vi "2nd head(json).vi"(11 "value":string[](array[string])=["@secondNumber@", "@itemName@", "@startTime@", "@stopTime@", "@secondResult@"]) -> (3 "midVar_Content":string)   [LabVIEW 2011]
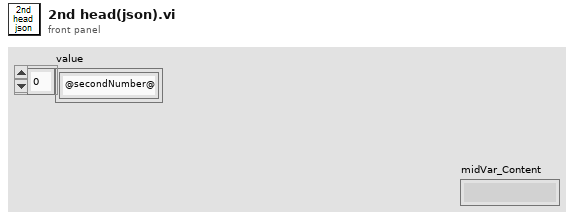
[diagram p1: front panel]
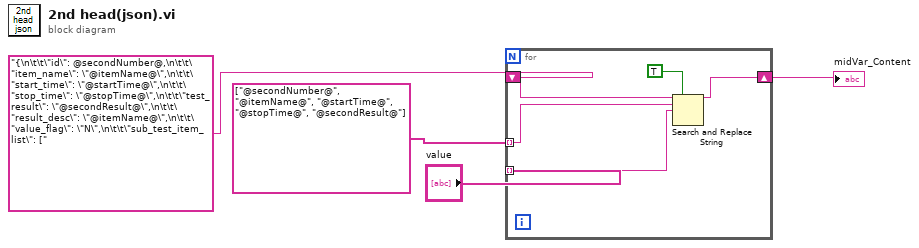
[diagram p0: block diagram]
diagram:
  n1 = for {
    tunnel: "value" -> [w5] mode=indexing
    tunnel: string[] ["@secondNumber@", "@itemName@", "@startTime@", "@stopTime@", "@secondResult@"] -> [w6] mode=indexing
    shift-right: [w8] -> w1
    shift-left: "{\n\t\t\"id\": @secondNumber@,\n\t\t\"item_name\": \"@itemName@\",\n\t\t\"start_time\": \"@startTime@\",\n\t\t\"stop_time\": \"@stopTime@\",\n\t\t\"test_result\": \"@secondResult@\",\n\t\t\"result_desc\": \"@itemName@\",\n\t\t\"value_flag\": \"N\",\n\t\t\"sub_test_item_list\": [" -> [w9]
    n2 = Search and Replace String(replace all?=TRUE ("替换全部？(F)"), input string=w9, search string=w6, replace string=w5) -> (result string=w8:string)  [unwired: 4 in, 3 out]
  }
  "midVar_Content" <- w1
